vi "Software Stop.vi"(8 "error in (no error)":errorcluster caption="错误输入（无错误）", 11 "UI 输入":refnum<class "UI.lvclass">) -> (0 "error out":errorcluster caption="错误输出", 3 "UI 输出":refnum<class "UI.lvclass">)   [LabVIEW 2019, in "UI.lvlib" / "UI.lvclass"]
uses:
  UI.lvclass
  C:/Program Files (x86)/National Instruments/LabVIEW 2019/vi.lib/ActorFramework/Actor/Actor.lvclass
  <vilib>/ActorFramework/Actor/Actor.lvclass/Actor.ctl
  <vilib>/ActorFramework/Message Enqueuer/Message Enqueuer.lvclass/Message Enqueuer.ctl
  UI.lvclass/UI.ctl
  <vilib>/ActorFramework/Message Enqueuer/Init from Existing Queue.vi
  <vilib>/ActorFramework/Message Enqueuer/Enqueue.vi
  C:/Program Files (x86)/National Instruments/LabVIEW 2019/vi.lib/ActorFramework/Message/Message.lvclass
  <vilib>/ActorFramework/Stop Msg/Stop Msg.lvclass
  <vilib>/ActorFramework/Message Priority Queue/Priority Enqueue.vi
  <vilib>/ActorFramework/Message Enqueuer/Message Enqueuer.lvclass
  Log/Log/Log.lvclass
  <vilib>/ActorFramework/Actor/Actor.lvclass
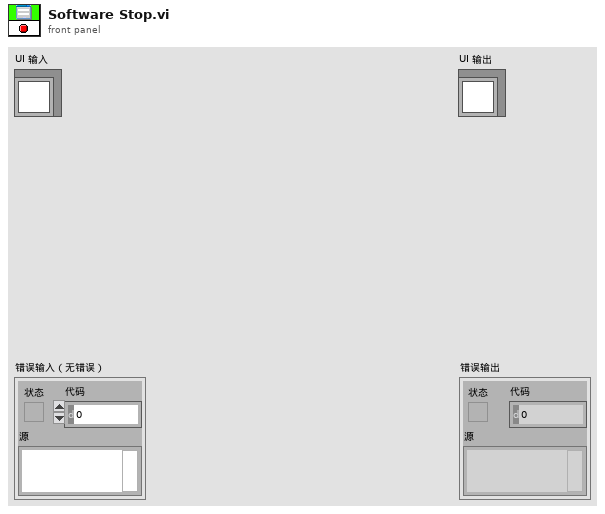
[diagram p1: front panel]
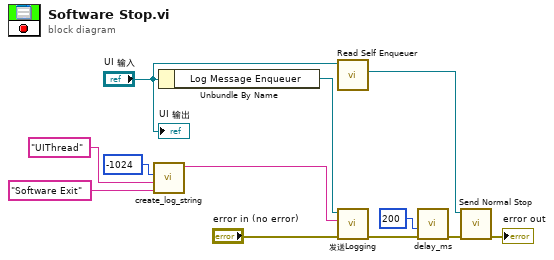
[diagram p0: block diagram]
diagram:
  n1 = call "create_log_string.vi"("source"="Software Exit" ("thread"), "thread"="UIThread", "Code"=-1024) -> ("log string"=w10:string)  [unwired: 8 in]
  n2 = Unbundle By Name("UI 输入") -> ("Log Message Enqueuer"=w12:refnum<class "Message Enqueuer.lvclass">)
  n3 = call <vilib>:"Read Self Enqueuer.vi"("Actor"="UI 输入") -> ("Self Enqueuer"=w3:refnum<class "Message Enqueuer.lvclass">)  [unwired: 10 in]
  n4 = call "发送Logging.vi"("error in (no error)"="error in (no error)", "Log"=w10, "Message Enqueuer"=w12) -> ("error out"=w11:errorcluster)  [unwired: 7 in, 1 out]
  n5 = call "delay_ms.vi"("error in (no error)"=w11, "delay time(ms)"=200) -> ("error out"=w5:errorcluster)  [unwired: 9 in]
  n6 = call <vilib>:"Send Normal Stop.vi"("error in (no error)"=w5, "Message Enqueuer"=w3) -> ("error out"=→"error out":errorcluster)  [unwired: 9 in]
  "UI 输出" <- "UI 输入"
